vi "PID Angle Correction.vi"(1 "Set angle":dbl, 2 "PID inputs":T3={"output range"={"high"=100.0, "low"=-100.0}, "PID gains"={"proportional gain (Kp)"=1.0, "integral time (Ki)"=0.0, "derivative time (Kd)"=0.0}, "Invert value"=FALSE} {"output range"."low" format="%.2f"; "output range"."high" format="%.2f"; "PID gains"."derivative time (Kd)" format="%.3f"; "PID gains"."integral time (Ki)" format="%.3f"; "PID gains"."proportional gain (Kp)" format="%.3f"}, 3 "PigeonIMUDevRef":T1={"DeviceStatus"={"status"=FALSE, "code"=0, "source"=""}, "Device Number"=21, "Type"=352321536, "Device ID"=352321557, "Handle"=23350768, "UsageFrame"=0, "Library Path"=path "libCTRE_PhoenixCCI.so"} {"Type" items=["CAN"=352321536, "TalonSRX"=33554432]}) -> (0 "Correction":dbl)   [LabVIEW 2023]
uses:
  <vilib>/Rock Robotics/WPI/ThirdParty/Phoenix-LabVIEW/Pigeon IMU/CTRE_PigeonIMU_DeviceRef.ctl
  <vilib>/Rock Robotics/WPI/ThirdParty/Phoenix-LabVIEW/Pigeon IMU/CTRE_PigeonIMU_ConnectionType.ctl
  <vilib>/Rock Robotics/WPI/ThirdParty/Phoenix-LabVIEW/Pigeon IMU/CTRE_PigeonIMU_GetYPR.vi
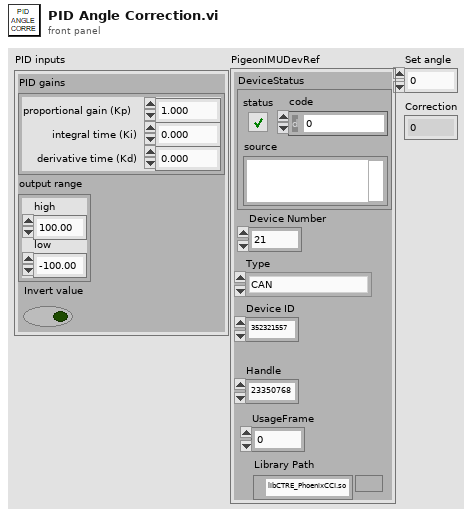
[diagram p1: front panel]
types:
  T1 = typedef "CTRE_PigeonIMU_DeviceRef.ctl" = cluster{"DeviceStatus":errorcluster, "Device Number":u8, "Type":T2, "Device ID":u32, "Handle":u64, "UsageFrame":u32, "Library Path":path}
  T2 = typedef "CTRE_PigeonIMU_ConnectionType.ctl" = u32
  T3 = cluster{"output range":cluster{"high":dbl, "low":dbl}, "PID gains":cluster{"proportional gain (Kp)":dbl, "integral time (Ki)":dbl, "derivative time (Kd)":dbl}, "Invert value":bool}
  T4 = cluster{"proportional gain (Kp)":dbl, "integral time (Ki)":dbl, "derivative time (Kd)":dbl}
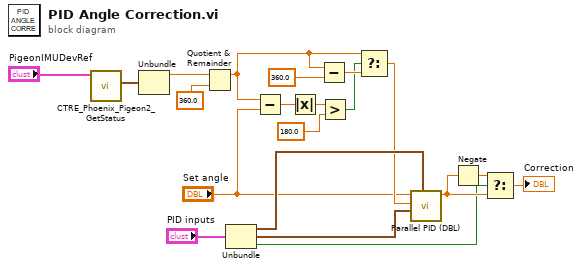
[diagram p0: block diagram]
diagram:
  n1 = call-poly <vilib>:"CTRE_Phoenix_Pigeon2_GetStatus.vi"("PigeonIMUDevRef"="PigeonIMUDevRef") -> ("Yaw Pitch Roll"=w13:cluster{"Yaw":dbl, "Pitch":dbl, "Roll":dbl})  [unwired: 8 in, 2 out]
  n2 = Unbundle(w13) -> ("Yaw"=w11:dbl)  [unwired: 2 out]
  n3 = Quotient & Remainder(x=w11, y=360.0) -> (x-y*floor(x/y)=w5:dbl)  [unwired: 1 out]
  n4 = Unbundle("PID inputs") -> ("output range"=w16:cluster{"high":dbl, "low":dbl}, "PID gains"=w15:T4, "Invert value"=w14:bool)
  n5 = Subtract(x=w5, y="Set angle") -> (x-y=w9:dbl)
  n6 = Absolute Value(x=w9) -> (abs(x)=w8:dbl)
  n7 = Subtract(x=w5, y=360.0) -> (x-y=w6:dbl)
  n8 = Greater?(x=w8, y=180.0) -> (0:w3:bool)
  n9 = Select(t=w5, s=w3, f=w6) -> (s? t:f=w2:dbl)
  n10 = call <vilib>:"Parallel PID (DBL).vi"("output range"=w16, "PID gains"=w15, "process variable"=w2, "setpoint"="Set angle") -> ("output"=w18:dbl)  [unwired: 4 in, 3 out]
  n11 = Negate(x=w18) -> (-x=w19:dbl)
  n12 = Select(t=w19, s=w14, f=w18) -> (s? t:f=→"Correction":dbl)
